vi "HFRR ADV v02.vi"() -> ()   [LabVIEW 2025] (continued)
                }
                frame 94 {
                  n3405 = local write "S 96"(w4363) -> ()
                }
                frame 95 {
                  n3406 = local write "S 97"(w4364) -> ()
                }
                frame 96 {
                  n3407 = local write "S 98"(w4365) -> ()
                }
                frame 97 {
                  n3408 = local write "S 99"(w4366) -> ()
                }
                frame 98 {
                  n3409 = local write "S 100"(w4367) -> ()
                }
                frame 99 {
                  n3410 = local write "S 101"(w4368) -> ()
                }
                frame 100 {
                  n3411 = local write "S 102"(w4369) -> ()
                }
                frame 101 {
                  n3412 = local write "S 103"(w4370) -> ()
                }
                frame 102 {
                  n3413 = local write "S 104"(w4371) -> ()
                }
                frame 103 {
                  n3414 = local write "S 105"(w4372) -> ()
                }
                frame 104 {
                  n3415 = local write "S 106"(w4373) -> ()
                }
                frame 105 {
                }
                frame 106 {
                  n3416 = property on="OK Button 17" class="Bool (strict)"("Boolean Text.Text"=w4374) -> ()  [unwired: 2 in, 2 out]
                }
                frame 107 {
                  n3417 = property on="OK Button 16" class="Bool (strict)"("Boolean Text.Text"=w4375) -> ()  [unwired: 2 in, 2 out]
                }
                frame 108 {
                  n3418 = property on="TITTLE" class="Str"("Caption.Text"=w4376) -> ()  [unwired: 2 in, 2 out]
                }
                frame 109 {
                  "String 30" <- w4377
                }
                frame 110 {
                  n3419 = property on="Test Date" class="Str"("Caption.Text"=w4378) -> ()  [unwired: 2 in, 2 out]
                  "String 31" <- w4378
                }
                frame 111 {
                  n3420 = property on="Sample ID" class="Str"("Caption.Text"=w4379) -> ()  [unwired: 2 in, 2 out]
                  "String 32" <- w4379
                }
                frame 112 {
                  n3421 = property on="Tested by" class="Str"("Caption.Text"=w4380) -> ()  [unwired: 2 in, 2 out]
                  "String 33" <- w4380
                }
                frame 113 {
                  n3422 = property on="System Configured Printers 2" class="Arr (strict)"("Caption.Text"=w4381) -> ()  [unwired: 2 in, 2 out]
                }
                frame 114 {
                  n3423 = property on="Selected Printer" class="Str"("Caption.Text"=w4382) -> ()  [unwired: 2 in, 2 out]
                }
                frame 115 {
                  n3424 = property on="Select Printer 3" class="DigNum (strict)"("Caption.Text"=w4383) -> ()  [unwired: 2 in, 2 out]
                }
                frame 116 {
                  n3425 = property on="Print" class="Bool (strict)"("Boolean Text.Text"=w4384) -> ()  [unwired: 2 in, 2 out]
                }
                frame 117 {
                  "String 41" <- w4385
                }
                frame 118 {
                  n3426 = property on="tested by" class="Str"("Caption.Text"=w4386) -> ()  [unwired: 2 in, 2 out]
                }
                frame 119 {
                }
                frame 120 {
                  n3427 = property on="Export" class="Bool (strict)"("Boolean Text.Text"=w4387) -> ()  [unwired: 2 in, 2 out]
                }
                frame 121 {
                }
                frame 122 {
                }
                frame 123 {
                  n3428 = property on="Select File Type" class="Enum (strict)"("Caption.Text"=w4390) -> ()  [unwired: 2 in, 2 out]
                }
                frame 124 {
                  n3429 = property on="s.NO" class="Str"("Caption.Text"=w4391) -> ()  [unwired: 2 in, 2 out]
                  "String 45" <- w4391
                }
                frame 125 {
                  n3430 = property on="trip1 8" class="Bool (strict)"("Boolean Text.Text"=w4392) -> ()  [unwired: 2 in, 2 out]
                }
                frame 126, Default {
                }
              }
            }
          }
          frame #1 {
            w4400 = TRUE ("Visible")
            n3431 = local read "S 91"() -> (w4417:string)
            n3432 = local read "S 90"() -> (w4416:string)
            n3433 = local read "S 88"() -> (w4415:string)
            n3434 = property on="File Path" class="Path"("Caption.Text"=w4416) -> ()  [unwired: 2 in, 2 out]
            n3435 = local read "S 71"() -> (w4410:string)
            n3436 = local read "S 86"() -> (w4412:string)
            n3437 = local read "S 85"() -> (w4413:string)
            n3438 = local read "S 87"() -> (w4411:string)
            n3439 = local read "S 84"() -> (w4414:string)
            n3440 = local read "S 103"() -> (w4399:string)
            n3441 = local read "S 104"() -> (w4398:string)
            n3442 = property on="Password" class="Str"("Caption.Text"=w4413) -> ()  [unwired: 2 in, 2 out]
            n3443 = property on="EDIT" class="Bool (strict)"("Boolean Text.Text"=w4410) -> ()  [unwired: 2 in, 2 out]
            n3444 = property on="SAVE" class="Bool (strict)"("Boolean Text.Text"=w4414) -> ()  [unwired: 2 in, 2 out]
            n3445 = Build Array(w4399, w4398) -> (w4397:string[])
            n3446 = property on="Heater Button" class="Bool (strict)"("Strings [4]"=w4397) -> ()  [unwired: 2 in, 2 out]
            n3447 = local read "S 92"() -> (w4409:string)
            n3448 = local read "S 93"() -> (w4408:string)
            n3449 = local read "S 105"() -> (w4395:string)
            n3450 = local read "S 106"() -> (w4394:string)
            n3451 = Build Array(w4409, w4408) -> ()  [unwired: 1 out]
            n3452 = Build Array(w4395, w4394) -> (w4396:string[])
            n3453 = local read "S 95"() -> (w4406:string)
            n3454 = local read "S 94"() -> (w4407:string)
            n3455 = local read "bs"() -> (w4422:string)
            n3456 = local read "as"() -> (w4423:string)
            n3457 = property on="Humidity" class="Bool (strict)"("Strings [4]"=w4396) -> ()  [unwired: 2 in, 2 out]
            n3458 = Concatenate Strings(w4422, "\r", w4423) -> ()  [unwired: 1 out]
            n3459 = property on="Rh After" class="DigNum (strict)"("Caption.Size to Text?"=TRUE ("Caption.Size to Text")) -> ()  [unwired: 2 in, 2 out]
            n3460 = local read "S 48"() -> (w4446:string)
            n3461 = local read "S 50"() -> (w4444:string)
            n3462 = local read "S 51"() -> (w4443:string)
            n3463 = local read "S 49"() -> (w4445:string)
            n3464 = local read "S 52"() -> (w4442:string)
            n3465 = local read "as"() -> (w4427:string)
            n3466 = local read "bs"() -> (w4428:string)
            n3467 = local read "S 56"() -> (w4441:string)
            n3468 = local read "S 57"() -> (w4440:string)
            n3469 = local read "S 58"() -> (w4439:string)
            n3470 = local read "S 59"() -> (w4438:string)
            n3471 = property on="OPEN" class="Bool (strict)"("Boolean Text.Text"=w4442) -> ()  [unwired: 2 in, 2 out]
            n3472 = property on="OPEN 1" class="Bool (strict)"("Boolean Text.Text"=w4446) -> ()  [unwired: 2 in, 2 out]
            n3473 = property on="OPEN 2" class="Bool (strict)"("Boolean Text.Text"=w4445) -> ()  [unwired: 2 in, 2 out]
            n3474 = property on="OPEN 3" class="Bool (strict)"("Boolean Text.Text"=w4444) -> ()  [unwired: 2 in, 2 out]
            n3475 = property on="OPEN 4" class="Bool (strict)"("Boolean Text.Text"=w4443) -> ()  [unwired: 2 in, 2 out]
            n3476 = Concatenate Strings(w4428, "\r", w4427) -> ()  [unwired: 1 out]
            n3477 = local read "S 102"() -> (w4401:string)
            n3478 = property on="КОФ1" class="DigNum (strict)"("Caption.Text"=w4441) -> ()  [unwired: 2 in, 2 out]
            n3479 = local read "S 98"() -> (w4405:string)
            n3480 = local read "S 99"() -> (w4404:string)
            n3481 = local read "S 100"() -> (w4403:string)
            n3482 = local read "S 101"() -> (w4402:string)
            n3483 = property on="КОФ2" class="DigNum (strict)"("Caption.Text"=w4440) -> ()  [unwired: 2 in, 2 out]
            n3484 = property on="КОФ3" class="DigNum (strict)"("Caption.Text"=w4439) -> ()  [unwired: 2 in, 2 out]
            n3485 = property on="КОФ4" class="DigNum (strict)"("Caption.Text"=w4438) -> ()  [unwired: 2 in, 2 out]
            n3486 = local read "bs"() -> (w4426:string)
            n3487 = local read "as"() -> (w4425:string)
            n3488 = local read "S 60"() -> (w4437:string)
            n3489 = local read "S 54"() -> (w4447:string)
            n3490 = Concatenate Strings(w4426, "\r", w4425) -> ()  [unwired: 1 out]
            n3491 = Concatenate Strings(w4447, w4437) -> ()  [unwired: 1 out]
            n3492 = local read "S 77"() -> (→"String 43":string)
            n3493 = local read "S 76"() -> (w4420:string)
            n3494 = local read "S 78"() -> (w4419:string)
            n3495 = local read "S 71"() -> (w4431:string)
            n3496 = local read "S 66"() -> (w4436:string)
            n3497 = local read "S 67"() -> (w4435:string)
            n3498 = local read "S 68"() -> (w4434:string)
            n3499 = local read "S 69"() -> (w4433:string)
            n3500 = local read "S 70"() -> (w4432:string)
            n3501 = property on="AIR TEMP" class="DigNum (strict)"("Caption.Text"=w4419) -> ()  [unwired: 2 in, 2 out]
            n3502 = property on="Set Strk" class="DigNum (strict)"("Caption.Text"=w4420) -> ()  [unwired: 2 in, 2 out]
            n3503 = property on="SPEED OUT:" class="DigNum (strict)"("Caption.Text"=w4434) -> ()  [unwired: 2 in, 2 out]
            n3504 = property on="EDIT" class="Bool (strict)"("Boolean Text.Text"=w4431) -> ()  [unwired: 2 in, 2 out]
            n3505 = local read "S 79"() -> (w4418:string)
          }
          frame #2 {
          }
        }
        n3506 = local write "Lan flag"(10.0 ("Lan flag")) -> ()
      }
      frame Enabled {
      }
    }
    n3507 = Wait (ms)(milliseconds to wait=u32 2000) -> ()  [unwired: 1 out]
    n3508 = local read "Quit"() -> (w4221:bool)
  }
  n3509 = while {
    shift-right: [w4453] -> _
    shift-left: _ -> [w4454]
    shift-right: [w4451] -> _
    shift-left: T18 {"Read Heave and Surge"="", "Bytes at Heave Port"=0.0, "Heave and Surge COM Port:"="COM9", "Com Port 2"="COM7", "Residual Due"="", "Heave COM Status 2"=TRUE, "Heave COM Status"=TRUE, "Port 2"=TRUE, "Sway PPR"=6400.0, "Surge PPR"=6400.0, "Heave PPR"=6400.0, "Sway Pitch"=2.0, "Surge Pitch"=3.0, "Heave Pitch"=4.0, "Sway Pulses/mm"=320.0, "Surge Pulses/mm"=1600.0, "Heave Pulses/mm"=1600.0, "inner loop"=0.0, "Read Heave and Surge 2"="", "String 36"="", "Write S"=FALSE, "WriteCC1"=[""], "Heave COM Loop"=0, "LastCom"="", "EXIT"=FALSE, "Error Heave"={"status"=TRUE, "code"=-1073807343, "source"=""}} -> [w4450]
    shift-right: [w4448] -> _
    shift-left: enum16{"init", "MAIN", "Panel Close"}."init" -> [w4449]
    stop <- w4452 stop-if-true
    # "HUMIDITY LOOP LOGIC"
    n3510 = case shown="\"MAIN\"" w4449 {
      tunnel: w4454 -> [w4468 w4493 w4594 w4596]
      tunnel: [w4463 w4477 w4594 w4596] -> w4453
      tunnel: [_ _ TRUE _] -> w4452
      tunnel: [w4460 w4478 w4592 w4595] -> w4451
      tunnel: w4450 -> [w4465 w4492 w4592 w4595]
      tunnel: [enum16{"init", "MAIN", "Panel Close"}."MAIN" w4487 _ _] -> w4448
      frame "init" {
        n3511 = local read "C3 :"() -> (w4455:refnum<visa-resource-name>)
        n3512 = Bundle By Name(cluster=w4465, "Heave and Surge COM Port:"=w4455) -> (w4464:T18)
        n3513 = call "Instrument fgv uno.vi"("Enum"=T32."INIT", "error in (no error) 2"=w4468, "INPUT"=w4464) -> ("error"=w4466:errorcluster, "output"=w4462:T18)  [unwired: 6 in, 1 out]
        n3514 = case shown="Error" w4466 {
          selector: w4466 -> [w4470 _]
          tunnel: [w4470 w4474] -> w4463
          tunnel: w4462 -> [w4469 w4472]
          tunnel: [w4469 w4471] -> w4461
          frame No Error {
          }
          frame Error {
            n3515 = call "Instrument fgv uno.vi"("Enum"=T32."ERROR INIT", "INPUT"=w4472) -> ("error"=w4475:errorcluster, "output"=w4471:T18)  [unwired: 7 in, 1 out]
            n3516 = call <vilib>:"Clear Errors.vi"("error in (no error)"=w4475) -> ("error out"=w4474:errorcluster)  [unwired: 5 in, 1 out]
          }
        }
        n3517 = local read "LastCom Humidity"() -> (w4458:string)
        n3518 = Unbundle By Name(w4461) -> ("Heave COM Status 2"=→"COM Status":bool, "Error Heave"=→"Error":errorcluster)  [unwired: 1 out]
        n3519 = Bundle By Name(cluster=w4461, "LastCom"=w4458) -> (w4460:T18)
      }
      frame "MAIN" {
        n3520 = Unbundle By Name(w4492) -> ("Com Port 2"=w4482:refnum<visa-resource-name>)
        n3521 = local read "C3 :"() -> (w4483:refnum<visa-resource-name>)
        n3522 = Bundle By Name(cluster=w4492, "Heave and Surge COM Port:"=w4483) -> (w4491:T18)
        n3523 = local write "COM Port Humidity :"(w4482) -> ()
        n3524 = Equal?(x=w4482, y=w4483) -> (x = y?=w4496:bool)
        n3525 = case shown="True" w4496 {
          tunnel: [w4536 w4553] -> w4481
          tunnel: w4493 -> [w4537 w4559]
          tunnel: w4491 -> [w4535 w4557]
          tunnel: [w4534 w4552] -> w4480
          frame False {
            n3526 = call <vilib>:"Clear Errors.vi"("error in (no error)"=w4537) -> ("error out"=w4533:errorcluster)  [unwired: 5 in, 1 out]
            n3527 = call "Instrument fgv uno.vi"("Enum"=T32."ERROR INIT", "error in (no error) 2"=w4533, "INPUT"=w4535) -> ("error"=w4539:errorcluster, "output"=w4534:T18)  [unwired: 6 in, 1 out]
            n3528 = call <vilib>:"Clear Errors.vi"("error in (no error)"=w4539) -> ("error out"=w4536:errorcluster)  [unwired: 5 in, 1 out]
          }
          frame True {
            n3529 = call "Instrument fgv uno.vi"("Enum"=T32."READ", "error in (no error) 2"=w4559, "INPUT"=w4557) -> ("error"=w4558:errorcluster, "output"=w4551:T18)  [unwired: 6 in, 1 out]
            n3530 = Bundle By Name(cluster=w4551, "String 36"="WRITE HUMIDITY") -> (w4550:T18)
            n3531 = case shown="True" "Write Humidity" {
              selector: "Write Humidity" -> [_ w4591]
              tunnel: w4558 -> [w4584 w4590]
              tunnel: [w4584 w4589] -> w4548
              tunnel: w4550 -> [w4583 w4587]
              tunnel: [w4583 w4586] -> w4547
              frame False {
              }
              frame True {
                n3532 = Not(x=w4591) -> (.not. x?=w4585:bool)
                n3533 = local write "Write Humidity"(w4585) -> ()
                n3534 = call "Instrument fgv uno.vi"("Enum"=T32."MANUAL WRITE", "error in (no error) 2"=w4590, "INPUT"=w4587) -> ("error"=w4589:errorcluster, "output"=w4586:T18)  [unwired: 6 in, 1 out]
              }
            }
            n3535 = call "Instrument fgv uno.vi"("Enum"=T32."WRITE", "error in (no error) 2"=w4548, "WriteCC1"="WriteHumidity", "INPUT"=w4547) -> ("error"=w4555:errorcluster, "WriteCC1"=w4541:string[], "output"=w4554:T18)  [unwired: 5 in]
            n3536 = Array Size(array="WriteHumidity") -> (size(s)=w4542:i32)
            n3537 = case shown="Error" w4555 {
              selector: w4555 -> [w4562 w4570]
              tunnel: w4554 -> [w4563 w4574]
              tunnel: [w4563 w4573] -> w4552
              tunnel: [w4562 w4571] -> w4553
              frame No Error {
              }
              frame Error {
                n3538 = Unbundle By Name(w4570) -> ("code"=w4566:i32)
                n3539 = Equal?(x=w4566, y=56) -> (x = y?=w4568:bool)
                n3540 = Equal?(x=w4566, y=-1073807339) -> (x = y?=w4564:bool)
                n3541 = Or(x=w4568, y=w4564) -> (x .or. y?=w4565:bool)
                n3542 = case shown="True" w4565 {
                  tunnel: w4574 -> [w4580 w4581]
                  tunnel: [w4579 w4581] -> w4573
                  tunnel: [w4578 w4582] -> w4572
                  tunnel: w4570 -> [w4575 w4582]
                  frame False {
                    n3543 = call <vilib>:"Clear Errors.vi"("error in (no error)"=w4575) -> ("error out"=w4576:errorcluster)  [unwired: 5 in, 1 out]
                    n3544 = call "Instrument fgv uno.vi"("Enum"=T32."ERROR INIT", "error in (no error) 2"=w4576, "INPUT"=w4580) -> ("error"=w4578:errorcluster, "output"=w4579:T18)  [unwired: 6 in, 1 out]
                  }
                  frame True {
                  }
                }
                n3545 = call <vilib>:"Clear Errors.vi"("error in (no error)"=w4572) -> ("error out"=w4571:errorcluster)  [unwired: 5 in, 1 out]
              }
            }
            n3546 = Greater Than 0?(x=w4542) -> (x > 0?=w4540:bool)
            n3547 = case shown="True" w4540 {
              tunnel: w4541 -> [_ w4561]
              frame False {
              }
              frame True {
                n3548 = local write "WriteHumidity"(w4561) -> ()
              }
            }
            n3549 = Unbundle By Name(w4552) -> ("LastCom"=→"LastCom Humidity":string, "Read Heave and Surge"=→"Read HUMIDITY":string)
          }
        }
        n3550 = Unbundle By Name(w4480) -> ("Heave COM Status 2"=w4495:bool, "Error Heave"=w4484:errorcluster, "Bytes at Heave Port"=→"Bytes at Humidity Port  2":dbl)  [unwired: 1 out]
        n3551 = disable-structure shown="Enabled" {
          disable-tunnel: w4481 -> [w4501 w4513]
          disable-tunnel: w4480 -> [w4500 w4514]
          disable-tunnel: [w4498 w4514] -> w4479
          disable-tunnel: [w4497 w4513] -> w4476
          frame Disabled {
            n3552 = local read "Humidity 2"() -> (w4499:bool)
            n3553 = case shown="True" w4499 {
              selector: w4499 -> [_ w4504]
              tunnel: w4501 -> [w4502 w4509]
              tunnel: [w4502 w4508] -> w4497
              tunnel: w4500 -> [w4503 w4507]
              tunnel: [w4503 w4506] -> w4498
              frame False {
              }
              frame True {
                n3554 = Not(x=w4504) -> (.not. x?=→"Humidity 2":bool)
                n3555 = call <vilib>:"Clear Errors.vi"("error in (no error)"=w4509) -> ("error out"=w4512:errorcluster)  [unwired: 5 in, 1 out]
                n3556 = call "Instrument fgv uno.vi"("Enum"=T32."ERROR INIT", "error in (no error) 2"=w4512, "INPUT"=w4507) -> ("error"=w4510:errorcluster, "output"=w4506:T18)  [unwired: 6 in, 1 out]
                n3557 = call <vilib>:"Clear Errors.vi"("error in (no error)"=w4510) -> ("error out"=w4508:errorcluster)  [unwired: 5 in, 1 out]
              }
            }
          }
          frame Enabled {
          }
        }
        n3558 = local write "Error"(w4484) -> ()
        n3559 = Unbundle By Name(w4484) -> ("status"=→"Humidity Port":bool)
        n3560 = Not(x=w4495) -> (.not. x?=w4485:bool)
        n3561 = local write "COM Status"(w4485) -> ()
        n3562 = case shown="Error .." w4476 {
          tunnel: w4479 -> [w4519 w4531]
          tunnel: w4476 -> [w4518 w4532]
          tunnel: [w4517 w4531] -> w4478
          tunnel: [w4516 w4532] -> w4477
          frame No Error {
            n3563 = First Call?() -> (First Call?: T/F=w4515:bool)
            n3564 = case shown="True" w4515 {
              tunnel: w4518 -> [w4520 w4527]
              tunnel: [w4520 w4526] -> w4516
              tunnel: w4519 -> [w4521 w4525]
              tunnel: [w4521 w4524] -> w4517
              frame False {
              }
              frame True {
                n3565 = call "Stall Data Flow.vim"("value in"=w4527, "milliseconds to wait"=u32 1000) -> ("value out"=w4523:errorcluster)  [unwired: 1 out]
                n3566 = call <vilib>:"Clear Errors.vi"("error in (no error)"=w4523) -> ("error out"=w4530:errorcluster)  [unwired: 5 in, 1 out]
                n3567 = call "Instrument fgv uno.vi"("Enum"=T32."ERROR INIT", "error in (no error) 2"=w4530, "INPUT"=w4525) -> ("error"=w4528:errorcluster, "output"=w4524:T18)  [unwired: 6 in, 1 out]
                n3568 = call <vilib>:"Clear Errors.vi"("error in (no error)"=w4528) -> ("error out"=w4526:errorcluster)  [unwired: 5 in, 1 out]
              }
            }
          }
          frame Error {
          }
        }
        n3569 = local read "Quit"() -> (w4488:bool)
        n3570 = Select(t=enum16{"init", "MAIN", "Panel Close"}."Panel Close", s=w4488, f=enum16{"init", "MAIN", "Panel Close"}."MAIN") -> (s? t:f=w4487:enum16{"init", "MAIN", "Panel Close"})
      }
      frame "Panel Close" {
      }
      frame Default {
      }
    }
  }
  n3571 = while {
    stop <- w4598 stop-if-true
    n3572 = call <vilib>:"High Resolution Polling Wait.vi"("seconds to wait"=0.05) -> ()  [unwired: 10 in, 1 out]
    n3573 = disable-structure shown="Enabled" {
      frame Disabled {
        n3574 = local read "Read HUMIDITY"() -> (w4599:string)
        n3575 = Spreadsheet String To Array(delimiter (Tab)=",", format string="", spreadsheet string=w4599, array type (2D Dbl)=string[] []) -> (array=w4618:string[])
        n3576 = for {
          tunnel: w4618 -> [w4627] mode=indexing
          tunnel: string[] ["STATE;", "SET;", "RH;", "T;", "AMB_RH;", "AMB_T;", "PUMP;", "FAN_IN;", "FAN_OUT;", "DEHUM;", "CURRENT;", "STALL;"] -> [w4626] mode=indexing
          tunnel: [w4625] -> w4617 mode=indexing
          n3577 = Match Pattern(string=w4627, regular expression=w4626) -> (after substring=w4625:string)  [unwired: 1 in, 3 out]
        }
        n3578 = Index Array(array=w4617) -> (element #1=w4616:string, element #2=w4615:string, element #3=w4607:string, element #4=w4606:string, element #5=w4605:string, element #6=w4614:string, element #7=w4613:string, element #8=w4612:string, element #9=w4611:string, element #10=w4610:string, element #11=w4609:string, element #12=w4608:string)  [unwired: 12 in]
        n3579 = Fract/Exp String To Number(string=w4607) -> (number=w4600:dbl)  [unwired: 3 in, 1 out]
        n3580 = Fract/Exp String To Number(string=w4605) -> (number=w4604:dbl)  [unwired: 3 in, 1 out]
        n3581 = local write "Ambient Humidity :"(w4604) -> ()
        n3582 = Equal?(x=w4600, y=0.0) -> (x = y?=w4602:bool)
        n3583 = case shown="True" w4602 {
          tunnel: [w4623 w4624] -> w4601
          tunnel: w4600 -> [w4623 _]
          frame False {
            (unwired) 0.0
            "Humidity temp" <- w4623
          }
          frame True {
            n3584 = local read "Humidity temp"() -> (w4624:dbl)
          }
        }
        "RH Numeric:" <- w4601
      }
      frame Enabled {
        n3585 = local read "Read HUMIDITY"() -> (w4647:string)
        n3586 = Spreadsheet String To Array(delimiter (Tab)=";", format string="", spreadsheet string=w4647, array type (2D Dbl)=dbl[] []) -> (array=w4643:dbl[])
        n3587 = Index Array(array=w4643) -> (element #1=→"STATE :":dbl, element #2=→"SET :":dbl, element #3=w4628:dbl, element #4=→"T :":dbl, element #5=→"AMB_RH :":dbl, element #6=→"AMB_T :":dbl, element #7=→"PUMP :":dbl, element #8=→"FAN_IN :":dbl, element #9=→"FAN_OUT :":dbl, element #10=→"DEHUM :":dbl, element #11=→"CURRENT :":dbl, element #12=→"STALL":dbl)  [unwired: 12 in]
        "RH :" <- w4628
        n3588 = Equal?(x=w4628, y=0.0) -> (x = y?=w4631:bool)
        n3589 = case shown="False" w4631 {
          tunnel: [w4648 w4649] -> w4632
          tunnel: w4628 -> [w4648 _]
          frame False {
            "Humidity temp 2" <- w4648
          }
          frame True {
            n3590 = local read "Humidity temp 2"() -> (w4649:dbl)
          }
        }
        n3591 = local write "RH Numeric:"(w4632) -> ()
      }
    }
    n3592 = local read "Quit"() -> (w4598:bool)
  }
  n3593 = while {
    shift-right: [w4655] -> _
    shift-left: _ -> [w4656]
    shift-right: [w4653] -> _
    shift-left: T20 {"Read Uno"="", "Bytes at Heave Port"=0.0, "UNO COM Port:"="COM9", "UNO COM Port: 2"="COM7", "Residual Due"="", "UNO COM Status 2"=TRUE, "UNO COM Status"=TRUE, "Port 2"=TRUE, "Sway PPR"=6400.0, "Surge PPR"=6400.0, "Heave PPR"=6400.0, "Sway Pitch"=2.0, "Surge Pitch"=3.0, "Heave Pitch"=4.0, "Sway Pulses/mm"=320.0, "Surge Pulses/mm"=1600.0, "Heave Pulses/mm"=1600.0, "inner loop"=0.0, "Read Heave and Surge 2"="", "String 36"="", "Write S"=FALSE, "WriteCC1"=[""], "Heave COM Loop"=0, "LastCom"="", "EXIT"=FALSE, "Error Heave"={"status"=TRUE, "code"=-1073807343, "source"=""}} -> [w4652]
    shift-right: [w4650] -> _
    shift-left: enum16{"init", "MAIN", "Panel Close"}."init" -> [w4651]
    stop <- w4654 stop-if-true
    # "UNO CODE LOGIC"
    n3594 = case shown="\"init\"" w4651 {
      tunnel: w4656 -> [w4670 w4693 w4763 w4765]
      tunnel: [w4665 w4679 w4763 w4765] -> w4655
      tunnel: [_ _ TRUE _] -> w4654
      tunnel: [w4661 w4678 w4761 w4764] -> w4653
      tunnel: w4652 -> [w4667 w4692 w4761 w4764]
      tunnel: [enum16{"init", "MAIN", "Panel Close"}."MAIN" w4687 _ _] -> w4650
      frame "init" {
        n3595 = local read "Com Port 1"() -> (w4657:refnum<visa-resource-name>)
        n3596 = Bundle By Name(cluster=w4667, "UNO COM Port:"=w4657) -> (w4666:T20)
        n3597 = call "Instrument fgv.vi"("Enum"=T32."INIT", "error in (no error) 2"=w4670, "INPUT"=w4666) -> ("error"=w4668:errorcluster, "output"=w4664:T18)  [unwired: 6 in, 1 out]
        n3598 = case shown="Error" w4668 {
          selector: w4668 -> [w4672 _]
          tunnel: [w4672 w4676] -> w4665
          tunnel: w4664 -> [w4671 w4674]
          tunnel: [w4671 w4673] -> w4662
          frame No Error {
          }
          frame Error {
            n3599 = call "Instrument fgv.vi"("Enum"=T32."ERROR INIT", "INPUT"=w4674) -> ("error"=w4677:errorcluster, "output"=w4673:T18)  [unwired: 7 in, 1 out]
            n3600 = call <vilib>:"Clear Errors.vi"("error in (no error)"=w4677) -> ("error out"=w4676:errorcluster)  [unwired: 5 in, 1 out]
          }
        }
        n3601 = local read "LastCom UNO"() -> (w4659:string)
        n3602 = Unbundle By Name(w4662) -> ("Heave COM Status 2"=→"Instrument Status":bool, "Error Heave"=→"Error  2":errorcluster)  [unwired: 1 out]
        n3603 = Bundle By Name(cluster=w4662, "LastCom"=w4659) -> (w4661:T18)
      }
      frame "MAIN" {
        n3604 = Unbundle By Name(w4692) -> ("UNO COM Port: 2"=w4682:refnum<visa-resource-name>)
        n3605 = local read "Com Port 1"() -> (w4683:refnum<visa-resource-name>)
        n3606 = local write "COM Port UNO :"(w4682) -> ()
        n3607 = Equal?(x=w4682, y=w4683) -> (x = y?=w4697:bool)
        n3608 = Bundle By Name(cluster=w4692, "UNO COM Port:"=w4683) -> (w4691:T20)
        n3609 = case shown="True" w4697 {
          tunnel: [w4717 w4734] -> w4681
          tunnel: w4693 -> [w4718 w4740]
          tunnel: w4691 -> [w4716 w4738]
          tunnel: [w4715 w4733] -> w4680
          frame False {
            n3610 = call <vilib>:"Clear Errors.vi"("error in (no error)"=w4718) -> ("error out"=w4714:errorcluster)  [unwired: 5 in, 1 out]
            n3611 = call "Instrument fgv.vi"("Enum"=T32."ERROR INIT", "error in (no error) 2"=w4714, "INPUT"=w4716) -> ("error"=w4720:errorcluster, "output"=w4715:T18)  [unwired: 6 in, 1 out]
            n3612 = call <vilib>:"Clear Errors.vi"("error in (no error)"=w4720) -> ("error out"=w4717:errorcluster)  [unwired: 5 in, 1 out]
          }
          frame True {
            n3613 = call "Instrument fgv.vi"("Enum"=T32."READ", "error in (no error) 2"=w4740, "INPUT"=w4738) -> ("error"=w4739:errorcluster, "output"=w4732:T18)  [unwired: 6 in, 1 out]
            n3614 = Bundle By Name(cluster=w4732, "String 36"="WRITE UNO") -> (w4731:T18)
            n3615 = case shown="True" "Write" {
              selector: "Write" -> [_ w4755]
              tunnel: w4739 -> [w4753 w4760]
              tunnel: [w4753 w4759] -> w4729
              tunnel: w4731 -> [w4752 w4757]
              tunnel: [w4752 w4756] -> w4728
              frame False {
              }
              frame True {
                n3616 = Not(x=w4755) -> (.not. x?=w4754:bool)
                n3617 = local write "Write"(w4754) -> ()
                n3618 = call "Instrument fgv.vi"("Enum"=T32."MANUAL WRITE", "error in (no error) 2"=w4760, "INPUT"=w4757) -> ("error"=w4759:errorcluster, "output"=w4756:T18)  [unwired: 6 in, 1 out]
              }
            }
            n3619 = Array Size(array="Write UNO") -> (size(s)=w4726:i32)
            n3620 = Greater Than 0?(x=w4726) -> (x > 0?=w4725:bool)
            n3621 = call "Instrument fgv.vi"("Enum"=T32."WRITE", "error in (no error) 2"=w4729, "WriteCC1"="Write UNO", "INPUT"=w4728) -> ("error"=w4736:errorcluster, "WriteCC1 2"=w4727:string[], "output"=w4735:T18)  [unwired: 5 in]
            n3622 = case shown="True" w4725 {
              tunnel: w4727 -> [_ w4742]
              frame False {
              }
              frame True {
                n3623 = local write "Write UNO"(w4742) -> ()
              }
            }
            n3624 = case shown="Error" w4736 {
              selector: w4736 -> [w4743 w4746]
              tunnel: w4735 -> [w4744 w4751]
              tunnel: [w4744 w4750] -> w4733
              tunnel: [w4743 w4748] -> w4734
              frame No Error {
              }
              frame Error {
                n3625 = call <vilib>:"Clear Errors.vi"("error in (no error)"=w4746) -> ("error out"=w4745:errorcluster)  [unwired: 5 in, 1 out]
                n3626 = call "Instrument fgv.vi"("Enum"=T32."ERROR INIT", "error in (no error) 2"=w4745, "INPUT"=w4751) -> ("error"=w4749:errorcluster, "output"=w4750:T18)  [unwired: 6 in, 1 out]
                n3627 = call <vilib>:"Clear Errors.vi"("error in (no error)"=w4749) -> ("error out"=w4748:errorcluster)  [unwired: 5 in, 1 out]
              }
            }
            n3628 = Unbundle By Name(w4733) -> ("LastCom"=→"LastCom UNO":string, "Read Heave and Surge"=→"Read UNO":string)
          }
        }
        n3629 = Unbundle By Name(w4680) -> ("Heave COM Status 2"=w4696:bool, "Heave COM Status"=w4686:bool, "Error Heave"=w4684:errorcluster, "Bytes at Heave Port"=→"Bytes at Uno":dbl)
        n3630 = Not(x=w4686) -> (.not. x?=w4694:bool)
        n3631 = Not(x=w4696) -> (.not. x?=w4685:bool)
        n3632 = local write "Instrument Status"(w4694) -> ()
        n3633 = local write "Error  2"(w4684) -> ()
        n3634 = local write "Port 1a"(w4686) -> ()
        n3635 = local read "Quit"() -> (w4688:bool)
        n3636 = local write "COM Status"(w4685) -> ()
        n3637 = Select(t=enum16{"init", "MAIN", "Panel Close"}."Panel Close", s=w4688, f=enum16{"init", "MAIN", "Panel Close"}."MAIN") -> (s? t:f=w4687:enum16{"init", "MAIN", "Panel Close"})
        n3638 = case shown="No Error" w4681 {
          tunnel: w4681 -> [w4701 w4713]
          tunnel: w4680 -> [w4700 w4712]
          tunnel: [w4699 w4713] -> w4679
          tunnel: [w4698 w4712] -> w4678
          frame No Error {
            n3639 = First Call?() -> (First Call?: T/F=w4702:bool)
            n3640 = case shown="True" w4702 {
              tunnel: w4700 -> [w4704 w4711]
              tunnel: [w4704 w4710] -> w4698
              tunnel: [w4703 w4708] -> w4699
              tunnel: w4701 -> [w4703 w4705]
              frame False {
              }
              frame True {
                n3641 = call <vilib>:"Clear Errors.vi"("error in (no error)"=w4705) -> ("error out"=w4706:errorcluster)  [unwired: 5 in, 1 out]
                n3642 = call "Instrument fgv.vi"("Enum"=T32."ERROR INIT", "error in (no error) 2"=w4706, "INPUT"=w4711) -> ("error"=w4709:errorcluster, "output"=w4710:T18)  [unwired: 6 in, 1 out]
                n3643 = call <vilib>:"Clear Errors.vi"("error in (no error)"=w4709) -> ("error out"=w4708:errorcluster)  [unwired: 5 in, 1 out]
              }
            }
          }
          frame Error {
          }
        }
      }
      frame "Panel Close" {
      }
      frame Default {
      }
    }
  }
